vi "PrepandSignItemsNames.vi"(11 "VI Data in":T1[](array[typedef])) -> (3 "Array":string[](array[string]))   [LabVIEW 2016, in "update vi properties.lvlib"]
uses:
  update vi properties.lvlib
  Cluster_Data.ctl
  <vilib>/picture/picture.llb/imagedata.ctl
panel:
  # "Connector Pane"
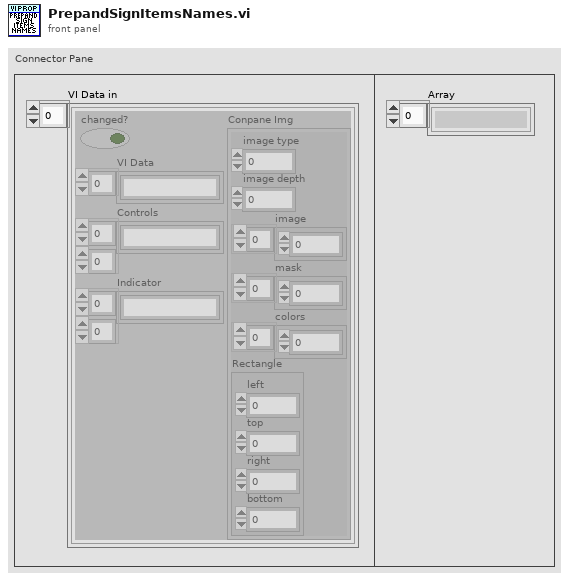
[diagram p1: front panel]
types:
  T1 = typedef "update vi properties.lvlib/Cluster_Data.ctl" = cluster{"changed?":bool, "VI Data":string[], "Controls":string[][], "Indicator":string[][], "Conpane Img":T2}
  T2 = typedef "imagedata.ctl" = cluster{"image type":i32, "image depth":i32, "image":u8[], "mask":u8[], "colors":u32[], "Rectangle":cluster{"left":i16, "top":i16, "right":i16, "bottom":i16}}
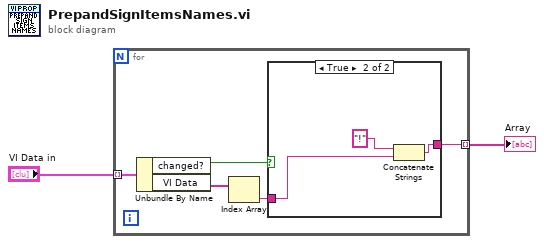
[diagram p0: block diagram]
diagram:
  n1 = for {
    tunnel: "VI Data in" -> [w7] mode=indexing
    tunnel: [w5] -> w2 mode=indexing
    n2 = Unbundle By Name(w7) -> ("changed?"=w3:bool, "VI Data"=w6:string[])
    n3 = Index Array(array=w6) -> (element=w4:string)  [unwired: 1 in]
    n4 = case shown="True" w3 {
      tunnel: [w8 w11] -> w5
      tunnel: w4 -> [w8 w10]
      frame False {
      }
      frame True {
        n5 = Concatenate Strings("!" ("format string"), w10) -> (w11:string)
      }
    }
  }
  "Array" <- w2
